vi "标定授权全局.vi"() -> ()   [LabVIEW 2013]
panel:
  out "功能解锁码":u8
  out "写其它参数":bool
  out "写SOC":bool
  in  "解锁类型":enum16{"读取", "写", "下载"}(ring)
  out "CTR":u8
  out "key":u32
  out "true":bool
  out "错误":bool
  out "连接状态":bool=TRUE
  out "读取相关功能":bool
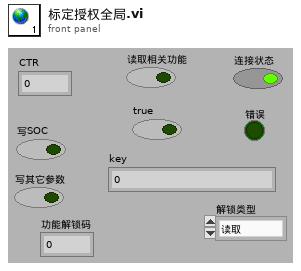
[diagram p1: front panel]
diagram:
